vi "Database_search.vi"() -> ()   [LabVIEW 2021]
doc: "This VI search the data in the data base."
uses:
  Acc-data-array-of-cluster.ctl
  Search_option.ctl
panel:
  in  "Stop":bool
  out "Valid Upto Search Result":T1[](array[typedef])
  out "Card Number Search Result":T1
  out "Card Holder Name Search result":T1[](array[typedef])
  out "Search Time (ms)":dbl
  in  "Search Option":T2
  in  "Valid Upto":dbl=2010.0 min=2000.0 max=2065.0 step=1.0
  in  "Card Number":dbl
  in  "Card Holder Name":string
  in  "Array":T1[](array[typedef])
  # "DATA BASE"
  # "SEARCH BOX"
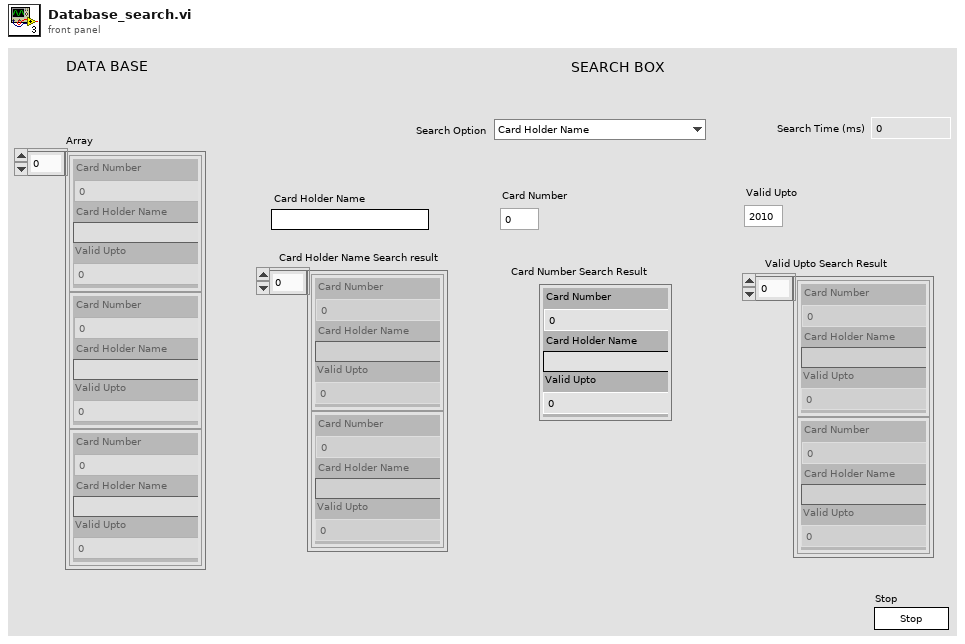
[diagram p1: front panel]
types:
  T1 = typedef "Acc-data-array-of-cluster.ctl" = cluster{"Card Number":dbl, "Valid Upto":dbl, "Card Holder Name":string}
  T2 = typedef "Search_option.ctl" = enum16{"Card Holder Name ", "Card Number", "Valid Upto"}
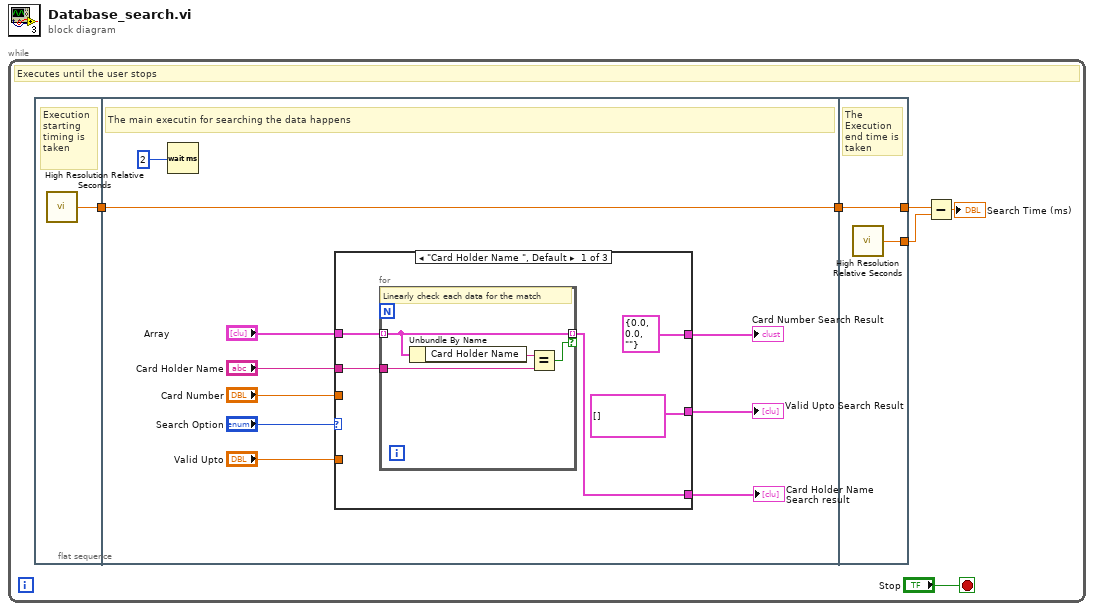
[diagram p0: block diagram]
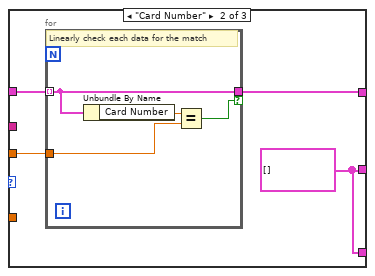
[diagram p2: hidden frame]
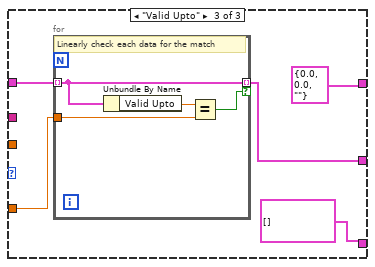
[diagram p3: hidden frame]
diagram:
  n1 = while {
    stop <- "Stop" stop-if-true
    # "Executes until the user stops"
    n2 = flat-sequence {
      tunnel: [w7] -> w6
      tunnel: w6 -> [w10]
      tunnel: [w10] -> w1
      tunnel: [w44] -> w4
      tunnel: [w45] -> w5
      tunnel: w1 -> [w45]
      frame #0 {
        # "Execution starting timing is  taken"
        n3 = call <vilib>:"High Resolution Relative Seconds.vi"() -> ("relative seconds"=w7:dbl)
      }
      frame #1 {
        # "The main executin for searching the data happens"
        n4 = Wait (ms)(milliseconds to wait=u32 2) -> ()  [unwired: 1 out]
        n5 = case shown="\"Card Holder Name \", Default" "Search Option" {
          tunnel: "Array" -> [w22 w28 w39]
          tunnel: "Card Number" -> [_ w30 _]
          tunnel: [T1 {"Card Number"=0.0, "Valid Upto"=0.0, "Card Holder Name"=""} ("Account Details") w29 T1 {"Card Number"=0.0, "Valid Upto"=0.0, "Card Holder Name"=""} ("Account Details")] -> w8
          tunnel: "Card Holder Name" -> [w21 _ _]
          tunnel: [w20 w27 T1[] [] ("Array")] -> w13
          tunnel: "Valid Upto" -> [_ _ w38]
          tunnel: [T1[] [] ("Array") w27 w37] -> w11
          frame "Card Holder Name ", Default {
            n6 = for {
              tunnel: [w24] -> w20 mode=indexing if=w25
              tunnel: w22 -> [w24] mode=indexing
              tunnel: w21 -> [w23]
              # "Linearly check each data for the match"
              n7 = Unbundle By Name(w24) -> ("Card Holder Name"=w26:string)
              n8 = Equal?(x=w26, y=w23) -> (x = y?=w25:bool)
            }
          }
          frame "Card Number" {
            w27 = T1[] [] ("Array")
            n9 = for {
              tunnel: w30 -> [w33]
              tunnel: [w31] -> w29 if=w32
              tunnel: w28 -> [w31] mode=indexing
              # "Linearly check each data for the match"
              n10 = Unbundle By Name(w31) -> ("Card Number"=w34:dbl)
              n11 = Equal?(x=w34, y=w33) -> (x = y?=w32:bool)
            }
          }
          frame "Valid Upto" {
            n12 = for {
              tunnel: [w41] -> w37 mode=indexing if=w42
              tunnel: w39 -> [w41] mode=indexing
              tunnel: w38 -> [w40]
              # "Linearly check each data for the match"
              n13 = Unbundle By Name(w41) -> ("Valid Upto"=w43:dbl)
              n14 = Equal?(x=w43, y=w40) -> (x = y?=w42:bool)
            }
          }
        }
        "Card Holder Name Search result" <- w13
        "Card Number Search Result" <- w8
        "Valid Upto Search Result" <- w11
      }
      frame #2 {
        # "The Execution end time is taken"
        n15 = call <vilib>:"High Resolution Relative Seconds.vi"() -> ("relative seconds"=w44:dbl)
      }
    }
    n16 = Subtract(x=w5, y=w4) -> (x-y=→"Search Time (ms)":dbl)
  }
